vi "Read Enqueuer.vi"(8 "error in (no error)":errorcluster, 11 "[V] User List in":refnum<class "[V] User List.lvclass">) -> (0 "error out":errorcluster, 3 "[V] User List out":refnum<class "[V] User List.lvclass">)   [LabVIEW 2020, in "[V] User List.lvlib" / "[V] User List.lvclass"]
uses:
  [V] User List.lvclass
  C:/Program Files (x86)/National Instruments/LabVIEW 2020/vi.lib/ActorFramework/Actor/Actor.lvclass
  <vilib>/ActorFramework/Actor/Actor.lvclass/Actor.ctl
  <vilib>/ActorFramework/Message Enqueuer/Message Enqueuer.lvclass/Message Enqueuer.ctl
  [V] User List.lvclass/[V] User List.ctl
  <vilib>/ActorFramework/Message Enqueuer/Init from Existing Queue.vi
  <vilib>/ActorFramework/Message Enqueuer/Message Enqueuer.lvclass
  <vilib>/ActorFramework/Actor/Actor.lvclass
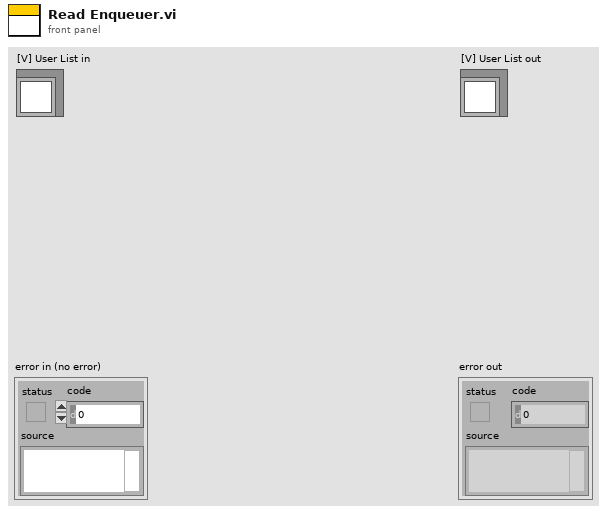
[diagram p1: front panel]
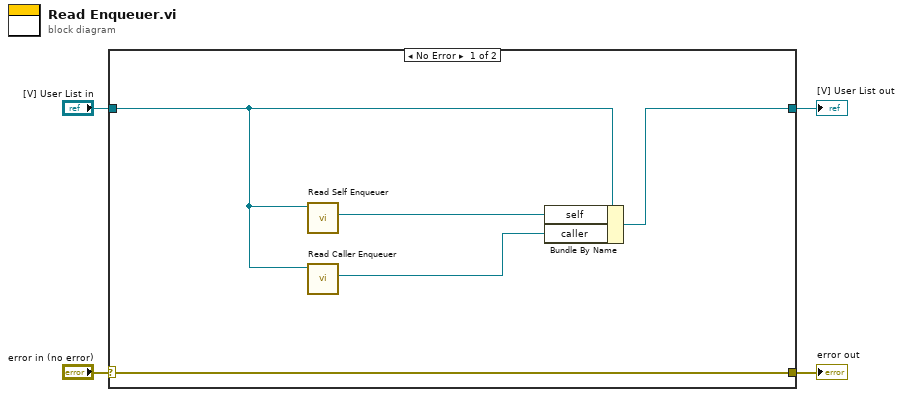
[diagram p0: block diagram]
diagram:
  n1 = case shown="No Error" "error in (no error)" {
    selector: "error in (no error)" -> [w9 w11]
    tunnel: [w9 w11] -> w3
    tunnel: [w5 w10] -> w1
    tunnel: "[V] User List in" -> [w6 w10]
    frame No Error {
      n2 = call <vilib>:"Read Self Enqueuer.vi"("Actor"=w6) -> ("Self Enqueuer"=w7:refnum<class "Message Enqueuer.lvclass">)  [unwired: 10 in]
      n3 = call <vilib>:"Read Caller Enqueuer.vi"("Actor"=w6) -> ("Caller Enqueuer"=w8:refnum<class "Message Enqueuer.lvclass">)  [unwired: 10 in]
      n4 = Bundle By Name(cluster=w6, "self"=w7, "caller"=w8) -> (w5:refnum<class "[V] User List.lvclass">)
    }
    frame Error {
    }
  }
  "error out" <- w3
  "[V] User List out" <- w1
